vi "Simple Example 1.vi"() -> ()   [LabVIEW 2014]
panel:
  in  "Error In":errorcluster
  # "This example is still in development."
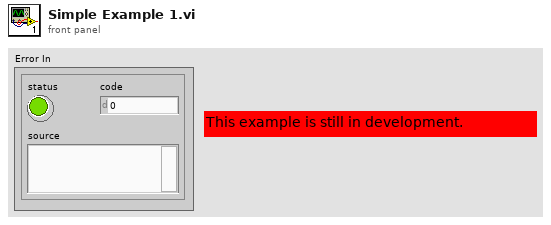
[diagram p1: front panel]
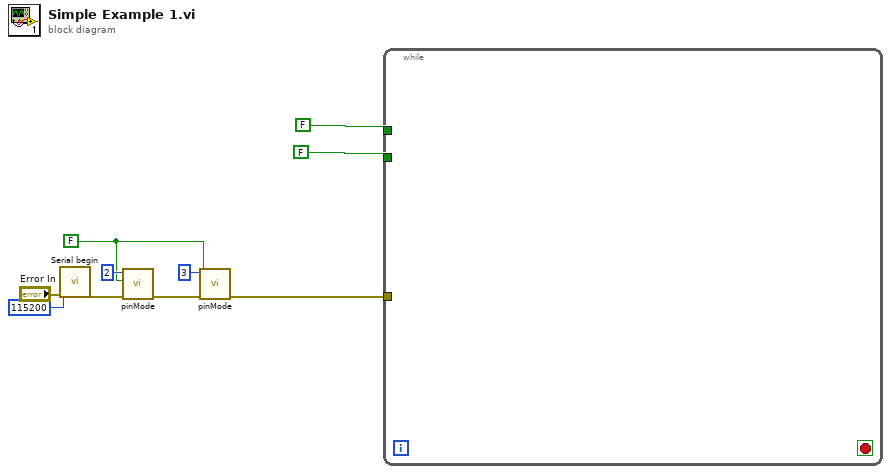
[diagram p0: block diagram]
diagram:
  w2 = FALSE ("output?")
  n1 = call <vilib>:"Serial begin.vi"("Error In"="Error In", "speed (Bd)"=115200) -> ("Error Out"=w5:errorcluster)  [unwired: 9 in]
  n2 = call <vilib>:"pinMode.vi"("Error In"=w5, "output?"=w2, "pin number"=2) -> ("Error Out"=w6:errorcluster)  [unwired: 8 in]
  n3 = call <vilib>:"pinMode.vi"("Error In"=w6, "output?"=w2, "pin number"=3) -> ("Error Out"=w1:errorcluster)  [unwired: 8 in]
  n4 = while {
    tunnel: FALSE -> [_]
    tunnel: FALSE -> [_]
    tunnel: w1 -> [_]
    stop <- _ stop-if-true
  }
